vi "ZF Login.vi"() -> ()   [LabVIEW 2021]
panel:
  in  "Tab Control":enum32{"Page 1", "Page 2"}(tab)
  in  "Enter Button":bool
  in  "Close":bool
  in  "Reset":bool
  in  "Login":bool
  in  "Password":string
  in  "User Name":string
  # "Welcome to ZF"
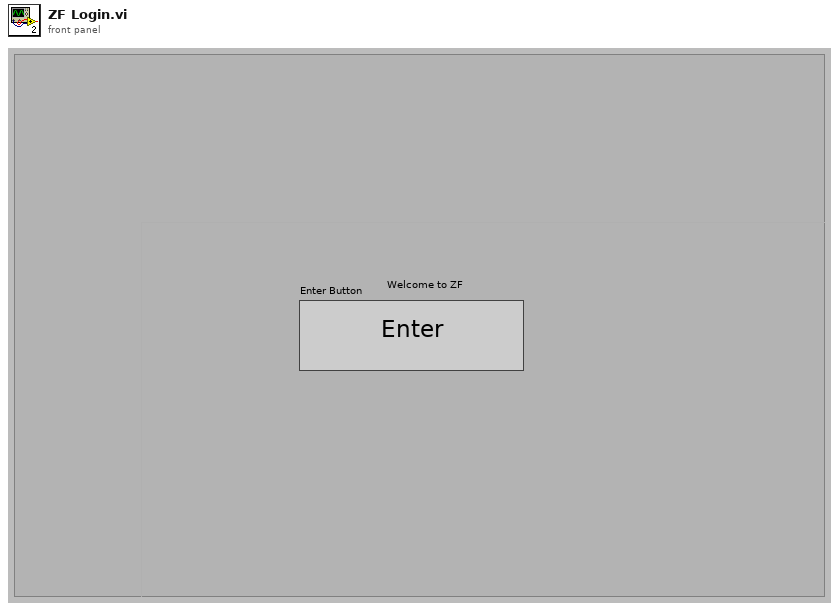
[diagram p1: front panel]
types:
  T1 = enum32{"Invalid", "Standard", "Closed", "Hidden", "Minimized", "Maximized"}
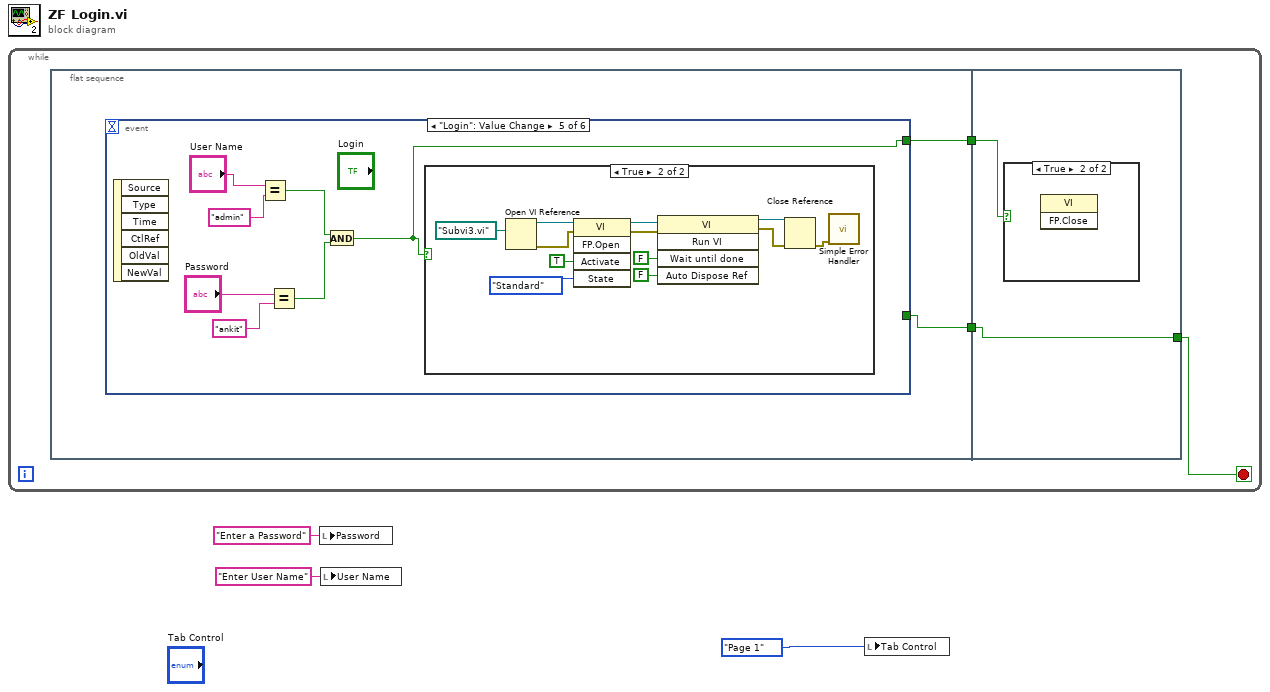
[diagram p0: block diagram]
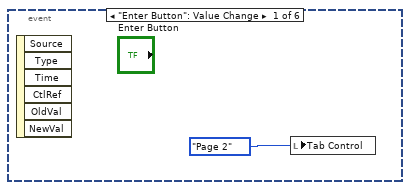
[diagram p2: hidden frame]
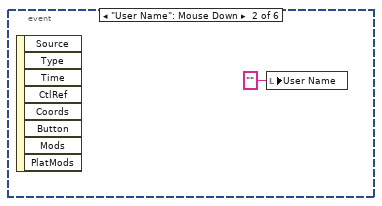
[diagram p3: hidden frame]
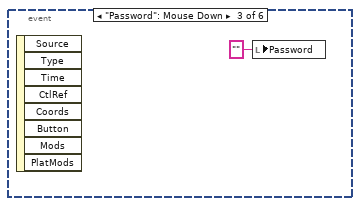
[diagram p4: hidden frame]
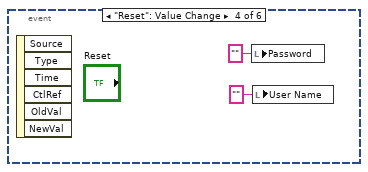
[diagram p5: hidden frame]
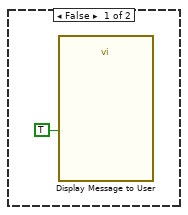
[diagram p6: hidden frame]
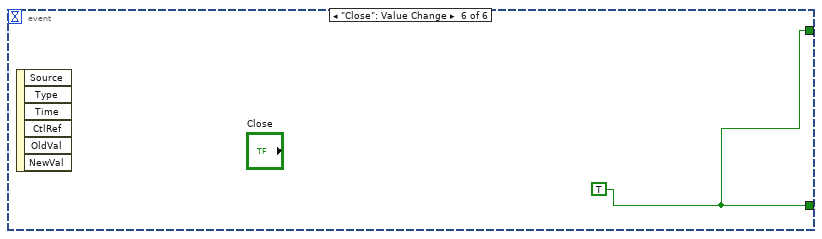
[diagram p7: hidden frame]
diagram:
  n1 = while {
    stop <- w4 stop-if-true
    n2 = flat-sequence {
      tunnel: [w8] -> w6
      tunnel: [w7] -> w5
      tunnel: w6 -> [w36]
      tunnel: w5 -> [w35]
      tunnel: [w35] -> w4
      frame #0 {
        n3 = event shown="[4] \"Login\": Value Change" {
          selector: _ -> [_ _ _ _ _ _]
          dyn-events: _ -> [_ _ _ _ _ _]
          timeout: _ -> [_ _ _ _ _ _]
          tunnel: [_ _ _ _ w14 w34] -> w8
          tunnel: [_ _ _ _ _ w34] -> w7
          event "Enter Button": Value Change {
            n4 = event-data() -> ()  [unwired: 1 in, 6 out]
            n5 = local write "Tab Control"(enum32{"Page 1", "Page 2"}."Page 2" ("Tab Control")) -> ()
          }
          event "User Name": Mouse Down {
            n6 = event-data() -> ()  [unwired: 1 in, 8 out]
            n7 = local write "User Name"("" ("User Name")) -> ()
          }
          event "Password": Mouse Down {
            n8 = event-data() -> ()  [unwired: 1 in, 8 out]
            n9 = local write "Password"("" ("Password")) -> ()
          }
          event "Reset": Value Change {
            n10 = event-data() -> ()  [unwired: 1 in, 6 out]
            n11 = local write "Password"("" ("Password")) -> ()
            n12 = local write "User Name"("" ("User Name")) -> ()
          }
          event "Login": Value Change {
            n13 = event-data() -> ()  [unwired: 1 in, 6 out]
            n14 = Equal?(x="User Name", y="admin") -> (x = y?=w16:bool)
            n15 = Equal?(x="Password", y="ankit") -> (x = y?=w15:bool)
            n16 = And(x=w16, y=w15) -> (x .and. y?=w14:bool)
            n17 = case shown="True" w14 {
              frame False {
                n18 = call "Display Message to User"("Enable"=TRUE) -> ()  [unwired: 9 in, 2 out]
              }
              frame True {
                n19 = Open VI Reference(vi path=path "Subvi3.vi") -> (vi reference=w32:refnum<vi>, error out=w29:errorcluster)  [unwired: 5 in]
                n20 = invoke class="VI" method="FP.Open"(reference=w32, error in=w29, "Activate"=TRUE ("Activate?"), "State"=T1."Standard") -> (reference out=w28:refnum<vi>, error out=w27:errorcluster)  [unwired: 1 in, 3 out]
                n21 = invoke class="VI" method="Run VI"(reference=w28, error in=w27, "Wait until done"=FALSE ("Wait Until Done"), "Auto Dispose Ref"=FALSE ("Auto Dispose Reference")) -> (reference out=w24:refnum<vi>, error out=w23:errorcluster)  [unwired: 1 in, 3 out]
                n22 = Close Reference(reference=w24, error in (no error)=w23) -> (error out=w22:errorcluster)
                n23 = call <vilib>:"Simple Error Handler.vi"("error in (no error)"=w22) -> ()  [unwired: 4 in, 5 out]
              }
            }
          }
          event "Close": Value Change {
            w34 = TRUE
            n24 = event-data() -> ()  [unwired: 1 in, 6 out]
          }
        }
      }
      frame #1 {
        n25 = case shown="True" w36 {
          frame False {
          }
          frame True {
            n26 = invoke class="VI" method="FP.Close"() -> ()  [unwired: 3 in, 3 out]
          }
        }
      }
    }
  }
  n27 = local write "Password"("Enter a Password" ("Password")) -> ()
  n28 = local write "User Name"("Enter User Name" ("User Name")) -> ()
  n29 = local write "Tab Control"(enum32{"Page 1", "Page 2"}."Page 1" ("Tab Control")) -> ()
